vi "Calibrate ISTR.vi"(7 "String":u8, 8 "error in (no error)":errorcluster, 9 "Position in":u32, 10 "Cree Comms in":refnum<class "Cree Communications.lvclass">, 11 "Calibration in":refnum<class "Calibration.lvclass">) -> (0 "error out":errorcluster, 1 "Position out":u32, 2 "Cree Comms out":refnum<class "Cree Communications.lvclass">, 3 "Calibration out":refnum<class "Calibration.lvclass">, 4 "Passed":bool, 6 "Fail Code":string)   [LabVIEW 2015, in "Calibration.lvclass"]
uses:
  Calibration.lvclass
  Classes/Cree Communications/Class/Cree Communications.lvclass
  Classes/Application/Class/Application.lvclass
  Test Class/Test Class.lvclass
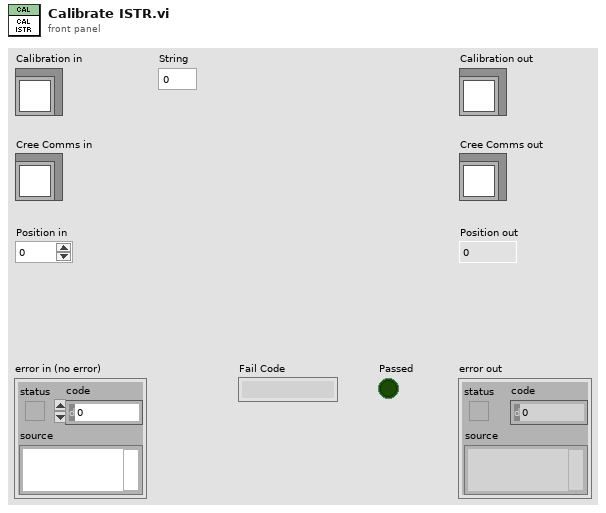
[diagram p1: front panel]
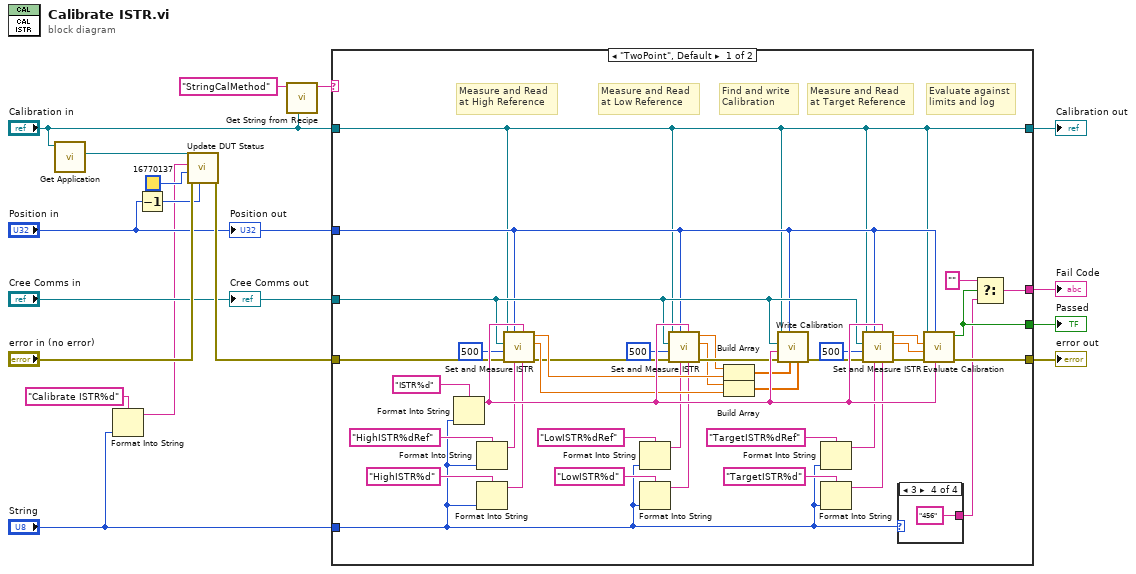
[diagram p0: block diagram]
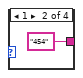
[diagram p3: hidden frame]
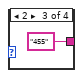
[diagram p4: hidden frame]
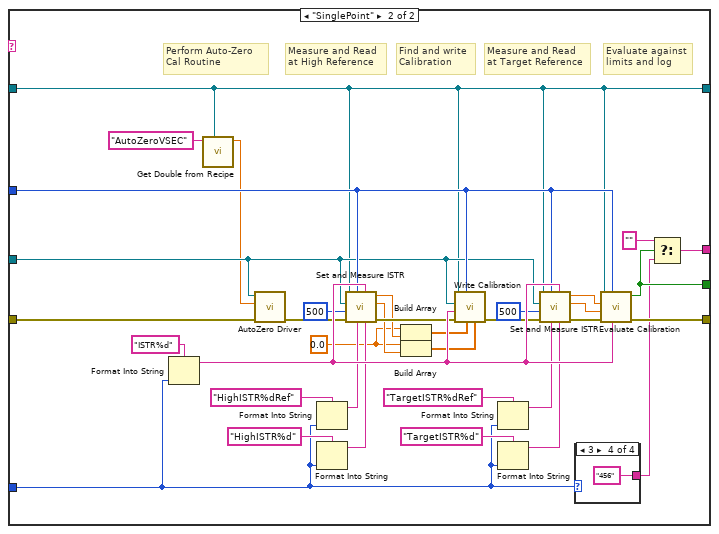
[diagram p5: hidden frame]
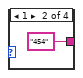
[diagram p7: hidden frame]
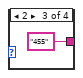
[diagram p8: hidden frame]
diagram:
  n1 = call "Get Application.vi"("Test Class in"="Calibration in") -> ("Application.lvlib:Application.lvclass"=w11:refnum<class "Application.lvclass">)  [unwired: 9 in, 1 out]
  n2 = Format Into String(format string="Calibrate ISTR%d" ("Calibration Type"), "String") -> (resulting string=w5:string)  [unwired: 2 in, 1 out]
  n3 = Decrement(x="Position in") -> (x-1=w9:u32)
  n4 = call "Update DUT Status.vi"("Position"=w9, "error in (no error)"="error in (no error)", "BG Color"=u32 16770137, "Message ('')"=w5, "Application in"=w11) -> ("error out"=w16:errorcluster)  [unwired: 5 in, 1 out]
  n5 = call "Get String from Recipe.vi"("Test Class in"="Calibration in", "Name"="StringCalMethod") -> ("Value"=w1:string)  [unwired: 7 in, 2 out]
  n6 = case shown="\"TwoPoint\", Default" w1 {
    tunnel: w16 -> [w55 w66]
    tunnel: [w51 w90] -> w15
    tunnel: [w50 w89] -> w14
    tunnel: [w48 w87] -> w13
    tunnel: "Cree Comms in" -> [w21 w64]
    tunnel: "Calibration in" -> [w18 w63]
    tunnel: "Position in" -> [w20 w70]
    tunnel: "String" -> [w19 w69]
    tunnel: [w18 w63] -> w4
    frame "TwoPoint", Default {
      # "Evaluate against\nlimits and log"
      # "Measure and Read\nat Target Reference"
      # "Find and write\nCalibration"
      # "Measure and Read\nat Low Reference"
      # "Measure and Read\nat High Reference"
      n7 = Format Into String(format string="ISTR%d" ("Calibration Type"), w19) -> (resulting string=w56:string)  [unwired: 2 in, 1 out]
      n8 = Format Into String(format string="HighISTR%dRef" ("Name"), w19) -> (resulting string=w38:string)  [unwired: 2 in, 1 out]
      n9 = Format Into String(format string="HighISTR%d" ("Name"), w19) -> (resulting string=w37:string)  [unwired: 2 in, 1 out]
      n10 = call "Set and Measure ISTR.vi"("Header"=w37, "String"=w56, "Name"=w38, "Position in"=w20, "error in (no error)"=w55, "Measurement Wait Time"=u32 500, "Cree Comms in"=w21, "Calibration in"=w18) -> ("error out"=w31:errorcluster, "DSpic Measurement"=w35:dbl, "Actual Measurement"=w36:dbl)  [unwired: 1 in]
      n11 = Format Into String(format string="LowISTR%dRef" ("Name"), w19) -> (resulting string=w33:string)  [unwired: 2 in, 1 out]
      n12 = Format Into String(format string="LowISTR%d" ("Name"), w19) -> (resulting string=w32:string)  [unwired: 2 in, 1 out]
      n13 = call "Set and Measure ISTR.vi"("Header"=w32, "String"=w56, "Name"=w33, "Position in"=w20, "error in (no error)"=w31, "Measurement Wait Time"=u32 500, "Cree Comms in"=w21, "Calibration in"=w18) -> ("error out"=w54:errorcluster, "DSpic Measurement"=w29:dbl, "Actual Measurement"=w30:dbl)  [unwired: 1 in]
      n14 = Build Array(w30, w36) -> (w52:dbl[])
      n15 = Build Array(w29, w35) -> (w53:dbl[])
      n16 = call "Write Calibration.vi"("DSPic Measurements"=w53, "Actual Measurements"=w52, "Position in"=w20, "error in (no error)"=w54, "Calibration Type"=w56, "Cree Comms in"=w21, "Calibration in"=w18) -> ("error out"=w26:errorcluster)  [unwired: 4 in]
      n17 = Format Into String(format string="TargetISTR%dRef" ("Name"), w19) -> (resulting string=w28:string)  [unwired: 2 in, 1 out]
      n18 = Format Into String(format string="TargetISTR%d" ("Name"), w19) -> (resulting string=w27:string)  [unwired: 2 in, 1 out]
      n19 = call "Set and Measure ISTR.vi"("Header"=w27, "String"=w56, "Name"=w28, "Position in"=w20, "error in (no error)"=w26, "Measurement Wait Time"=u32 500, "Cree Comms in"=w21, "Calibration in"=w18) -> ("error out"=w25:errorcluster, "DSpic Measurement"=w23:dbl, "Actual Measurement"=w24:dbl)  [unwired: 1 in]
      n20 = case shown="3" w19 {
        tunnel: [_ "454" "455" "456"] -> w40
        frame Default {
        }
        frame 1 {
        }
        frame 2 {
        }
        frame 3 {
        }
      }
      n21 = call "Evaluate Calibration.vi"("Calibration Type"=w56, "Position"=w20, "Error in"=w25, "DSPic Measurement"=w23, "Actual Measurement"=w24, "Calibration in"=w18) -> ("Error out"=w51:errorcluster, "Passed"=w50:bool)  [unwired: 4 in]
      n22 = Select(t="", s=w50, f=w40) -> (s? t:f=w48:string)
    }
    frame "SinglePoint" {
      w60 = 0.0
      # "Evaluate against\nlimits and log"
      # "Measure and Read\nat Target Reference"
      # "Find and write\nCalibration"
      # "Perform Auto-Zero\nCal Routine"
      # "Measure and Read\nat High Reference"
      n23 = Format Into String(format string="ISTR%d" ("Calibration Type"), w69) -> (resulting string=w94:string)  [unwired: 2 in, 1 out]
      n24 = call "Get Double from Recipe.vi"("Test Class in"=w63, "Name"="AutoZeroVSEC") -> ("Value"=w62:dbl)  [unwired: 7 in, 2 out]
      n25 = call "AutoZero Driver.vi"("error in (no error)"=w66, "AutoZero VSEC"=w62, "Cree Comms in"=w64) -> ("error out"=w65:errorcluster)  [unwired: 8 in]
      n26 = Format Into String(format string="HighISTR%dRef" ("Name"), w69) -> (resulting string=w79:string)  [unwired: 2 in, 1 out]
      n27 = Format Into String(format string="HighISTR%d" ("Name"), w69) -> (resulting string=w78:string)  [unwired: 2 in, 1 out]
      n28 = call "Set and Measure ISTR.vi"("Header"=w78, "String"=w94, "Name"=w79, "Position in"=w70, "error in (no error)"=w65, "Measurement Wait Time"=u32 500, "Cree Comms in"=w64, "Calibration in"=w63) -> ("error out"=w93:errorcluster, "DSpic Measurement"=w67:dbl, "Actual Measurement"=w68:dbl)  [unwired: 1 in]
      n29 = Build Array(w60, w68) -> (w91:dbl[])
      n30 = Build Array(w60, w67) -> (w92:dbl[])
      n31 = call "Write Calibration.vi"("DSPic Measurements"=w92, "Actual Measurements"=w91, "Position in"=w70, "error in (no error)"=w93, "Calibration Type"=w94, "Cree Comms in"=w64, "Calibration in"=w63) -> ("error out"=w75:errorcluster)  [unwired: 4 in]
      n32 = Format Into String(format string="TargetISTR%dRef" ("Name"), w69) -> (resulting string=w77:string)  [unwired: 2 in, 1 out]
      n33 = Format Into String(format string="TargetISTR%d" ("Name"), w69) -> (resulting string=w76:string)  [unwired: 2 in, 1 out]
      n34 = call "Set and Measure ISTR.vi"("Header"=w76, "String"=w94, "Name"=w77, "Position in"=w70, "error in (no error)"=w75, "Measurement Wait Time"=u32 500, "Cree Comms in"=w64, "Calibration in"=w63) -> ("error out"=w74:errorcluster, "DSpic Measurement"=w72:dbl, "Actual Measurement"=w73:dbl)  [unwired: 1 in]
      n35 = case shown="3" w69 {
        tunnel: [_ "454" "455" "456"] -> w81
        frame Default {
        }
        frame 1 {
        }
        frame 2 {
        }
        frame 3 {
        }
      }
      n36 = call "Evaluate Calibration.vi"("Calibration Type"=w94, "Position"=w70, "Error in"=w74, "DSPic Measurement"=w72, "Actual Measurement"=w73, "Calibration in"=w63) -> ("Error out"=w90:errorcluster, "Passed"=w89:bool)  [unwired: 4 in]
      n37 = Select(t="", s=w89, f=w81) -> (s? t:f=w87:string)
    }
  }
  "error out" <- w15
  "Calibration out" <- w4
  "Passed" <- w14
  "Fail Code" <- w13
  "Position out" <- "Position in"
  "Cree Comms out" <- "Cree Comms in"
